vi "rad_Read AppImage Properties.vi"(0 "AppImage Properties Path":path, 5 "error in (no error)":errorcluster) -> (14 "AppImage Properties":T1, 15 "Supported":bool, 16 "Current":bool, 17 "Older":bool, 18 "Newer":bool, 19 "error out":errorcluster)   [LabVIEW 2016]
uses:
  TypeDefs/rad_Application Image Properties.ctl
  TypeDefs/rad_FPGA Properties.ctl
  TypeDefs/rad_FPGA Flash Properties.ctl
  <vilib>/Utility/config.llb/Read Key (String).vi
  rad_Globals.vi
  <vilib>/Utility/config.llb/NI_LVConfig.lvlib
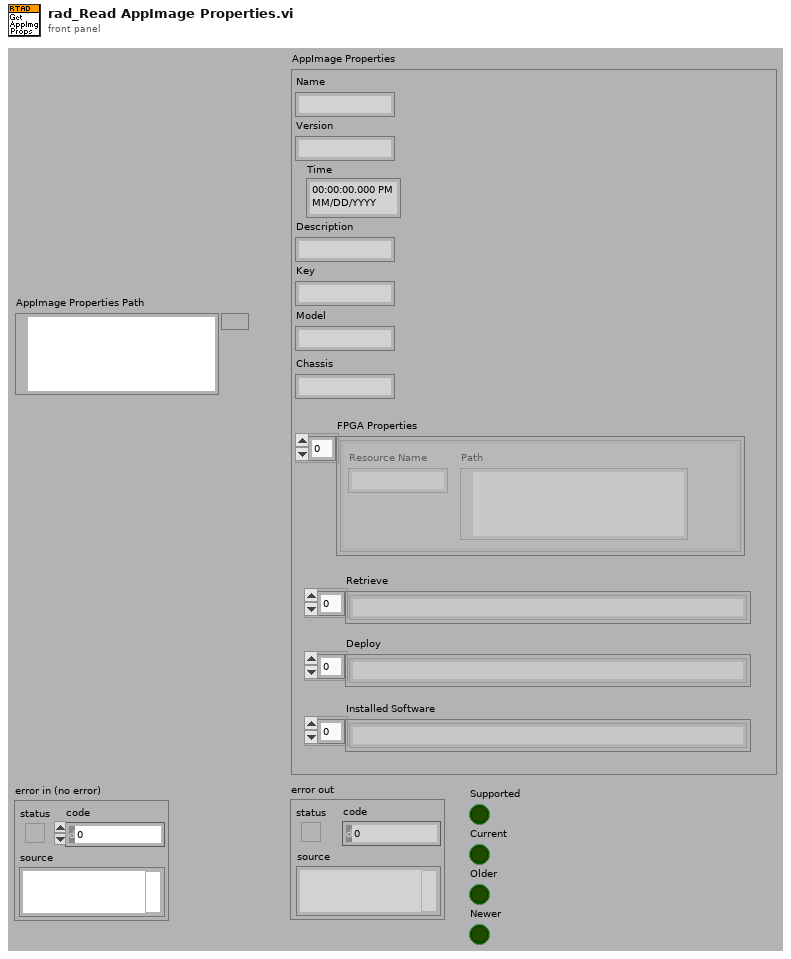
[diagram p1: front panel]
types:
  T1 = typedef "rad_Application Image Properties.ctl" = cluster{"Name":string, "Version":string, "Time":timestamp, "Description":string, "Key":string, "Chassis":string, "FPGA Properties":T2, "Model":string, "Retrieve":string[], "Deploy":string[], "Installed Software":string[]}
  T2 = typedef "rad_FPGA Properties.ctl" = T3[]
  T3 = typedef "rad_FPGA Flash Properties.ctl" = cluster{"Resource Name":string, "Path":path}
  T4 = typedef "NI_LVConfig.lvlib/Config Data RefNum.ctl" = refnum<k1>
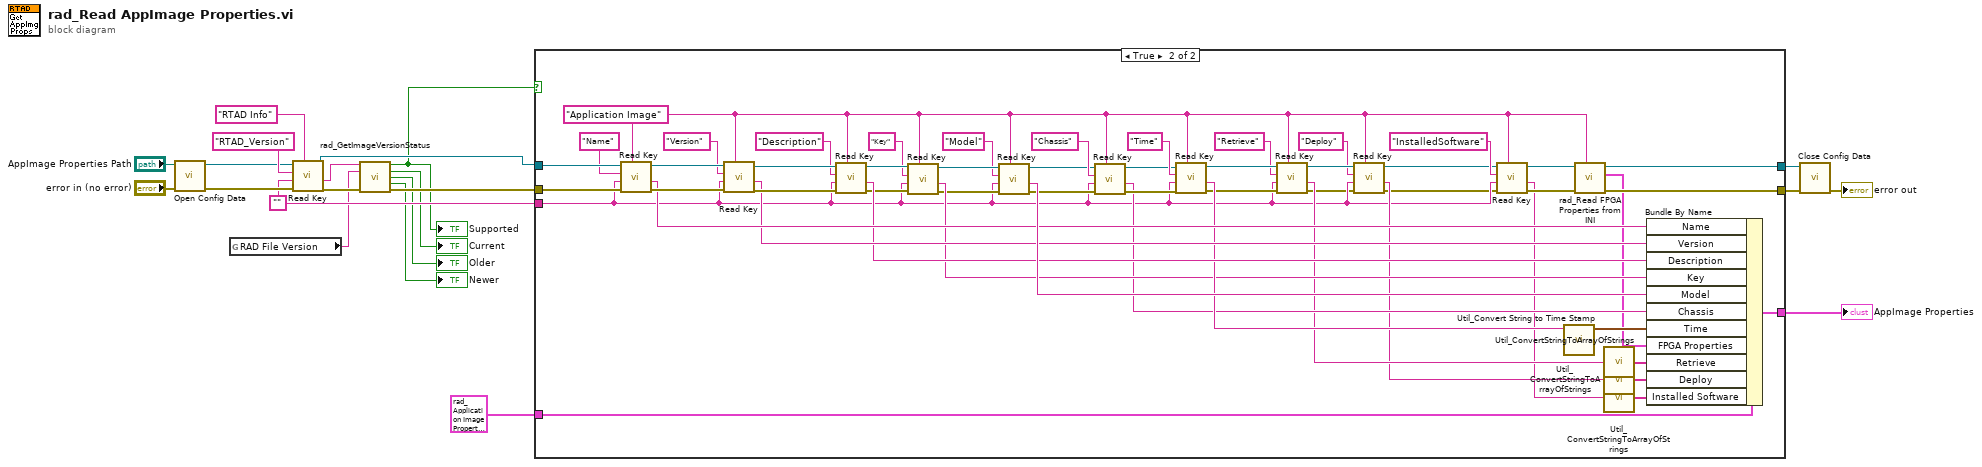
[diagram p0: block diagram]
diagram:
  w10 = ""
  n1 = call <vilib>:"Open Config Data.vi"("error in (no error)"="error in (no error)", "configuration file path"="AppImage Properties Path") -> ("error out"=w15:errorcluster, "refnum"=w16:T4)  [unwired: 7 in, 1 out]
  n2 = global read "rad_Globals.vi" "RAD File Version"() -> (w6:string)
  n3 = call-poly <vilib>:"Read Key.vi"("section"="RTAD Info", "error in (no error)"=w15, "default value"=w10, "key"="RTAD_Version", "refnum"=w16) -> ("error out"=w9:errorcluster, "value"=w7:string, "refnum out"=w18:T4)  [unwired: 1 in, 3 out]
  n4 = call "rad_GetImageVersionStatus.vi"("Image Version"=w7, "RAD Version"=w6, "error in (no error)"=w9) -> ("Supported"=w5:bool, "Current"=→"Current":bool, "Older"=→"Older":bool, "Newer"=→"Newer":bool, "error out"=w8:errorcluster)  [unwired: 8 in]
  "Supported" <- w5
  n5 = case shown="True" w5 {
    tunnel: w8 -> [w23 w76]
    tunnel: w18 -> [w24 w75]
    tunnel: [w22 w63] -> w13
    tunnel: [w24 w52] -> w12
    tunnel: [w23 w51] -> w11
    tunnel: w10 -> [_ w35]
    tunnel: T1 {"Name"="", "Version"="", "Time"=timestamp(0 s since 1904-01-01), "Description"="", "Key"="", "Chassis"="", "FPGA Properties"=[], "Model"="", "Retrieve"=[], "Deploy"=[], "Installed Software"=[]} ("AppImage Properties") -> [w22 w25]
    frame False {
    }
    frame True {
      w38 = "Application Image" ("section")
      n6 = call-poly <vilib>:"Read Key.vi"("section"=w38, "error in (no error)"=w76, "default value"=w35, "key"="Name", "refnum"=w75) -> ("error out"=w73:errorcluster, "value"=w67:string, "refnum out"=w72:T4)  [unwired: 1 in, 3 out]
      n7 = call-poly <vilib>:"Read Key.vi"("section"=w38, "error in (no error)"=w73, "default value"=w35, "key"="Version", "refnum"=w72) -> ("error out"=w71:errorcluster, "value"=w66:string, "refnum out"=w74:T4)  [unwired: 1 in, 3 out]
      n8 = call-poly <vilib>:"Read Key.vi"("section"=w38, "error in (no error)"=w71, "default value"=w35, "key"="Description", "refnum"=w74) -> ("error out"=w59:errorcluster, "value"=w65:string, "refnum out"=w60:T4)  [unwired: 1 in, 3 out]
      n9 = call-poly <vilib>:"Read Key.vi"("section"=w38, "error in (no error)"=w59, "default value"=w35, "key"="Key", "refnum"=w60) -> ("error out"=w47:errorcluster, "value"=w57:string, "refnum out"=w49:T4)  [unwired: 1 in, 3 out]
      n10 = call-poly <vilib>:"Read Key.vi"("section"=w38, "error in (no error)"=w47, "default value"=w35, "key"="Model", "refnum"=w49) -> ("error out"=w46:errorcluster, "value"=w77:string, "refnum out"=w48:T4)  [unwired: 1 in, 3 out]
      n11 = call-poly <vilib>:"Read Key.vi"("section"=w38, "error in (no error)"=w46, "default value"=w35, "key"="Chassis", "refnum"=w48) -> ("error out"=w55:errorcluster, "value"=w53:string, "refnum out"=w56:T4)  [unwired: 1 in, 3 out]
      n12 = call-poly <vilib>:"Read Key.vi"("section"=w38, "error in (no error)"=w55, "default value"=w35, "key"="Time", "refnum"=w56) -> ("error out"=w43:errorcluster, "value"=w61:string, "refnum out"=w44:T4)  [unwired: 1 in, 3 out]
      n13 = call-poly <vilib>:"Read Key.vi"("section"=w38, "error in (no error)"=w43, "default value"=w35, "key"="Retrieve", "refnum"=w44) -> ("error out"=w31:errorcluster, "value"=w40:string, "refnum out"=w32:T4)  [unwired: 1 in, 3 out]
      n14 = call-poly <vilib>:"Read Key.vi"("section"=w38, "error in (no error)"=w31, "default value"=w35, "key"="Deploy", "refnum"=w32) -> ("error out"=w26:errorcluster, "value"=w39:string, "refnum out"=w27:T4)  [unwired: 1 in, 3 out]
      n15 = call-poly <vilib>:"Read Key.vi"("section"=w38, "error in (no error)"=w26, "default value"=w35, "key"="InstalledSoftware", "refnum"=w27) -> ("error out"=w36:errorcluster, "value"=w33:string, "refnum out"=w37:T4)  [unwired: 1 in, 3 out]
      n16 = call "Util_Convert String to Time Stamp.vi"("Time"=w61) -> ("Time"=w62:timestamp)  [unwired: 10 out]
      n17 = call "rad_Read FPGA Properties from INI.vi"("section"=w38, "error in (no error)"=w36, "refnum in"=w37) -> ("error out"=w51:errorcluster, "FPGA Properties"=w50:T2, "refnum out"=w52:T4)  [unwired: 6 in]
      n18 = call "Util_ConvertStringToArrayOfStrings.vi"("String"=w40) -> ("Array<string>"=w42:string[])
      n19 = call "Util_ConvertStringToArrayOfStrings.vi"("String"=w39) -> ("Array<string>"=w41:string[])
      n20 = call "Util_ConvertStringToArrayOfStrings.vi"("String"=w33) -> ("Array<string>"=w34:string[])
      n21 = Bundle By Name(cluster=w25, "Name"=w67, "Version"=w66, "Description"=w65, "Key"=w57, "Model"=w77, "Chassis"=w53, "Time"=w62, "FPGA Properties"=w50, "Retrieve"=w42, "Deploy"=w41, "Installed Software"=w34) -> (w63:T1)
    }
  }
  "AppImage Properties" <- w13
  n22 = call <vilib>:"Close Config Data.vi"("error in (no error)"=w11, "refnum"=w12) -> ("error out"=→"error out":errorcluster)  [unwired: 1 in, 8 out]
